vi "Test_ConstructTransport_InvalidRefnum_Error.vi"(8 "error in (no error)":errorcluster, 11 "TestCase in":refnum<class "TestFormattedStringBinding.lvclass">) -> (0 "error out":errorcluster, 3 "TestCase out":refnum<class "TestFormattedStringBinding.lvclass">)   [LabVIEW 2017, in "TestFormattedStringBinding.lvclass"]
uses:
  TestFormattedStringBinding.lvclass
  Source/Concrete/FormattedStringBinding/FormattedStringBinding.lvclass/FormattedStringBinding.ctl
  Source/Concrete/FormattedStringBinding/FormattedStringBinding.lvclass
  C:/Git/composed-transport/Source/Concrete/TerminalValueBinding/TerminalValueBinding.lvclass
  <vilib>/Utility/error.llb/Error Cluster From Error Code.vi
  Source/Concrete/TerminalValueBinding/Construct Terminal Value Binding.vi
panel:
  out "Return Error":errorcluster
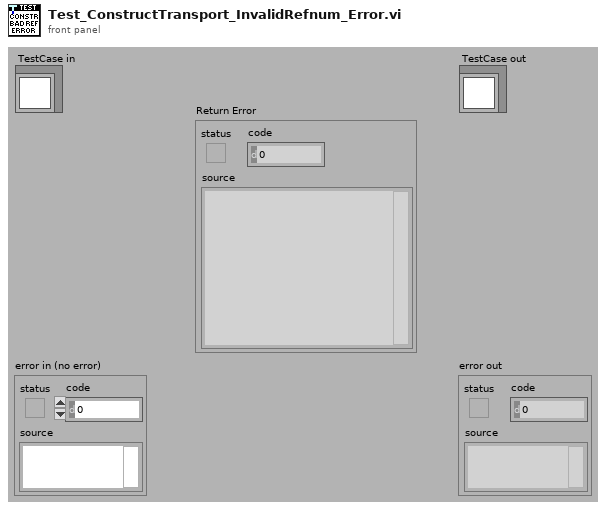
[diagram p1: front panel]
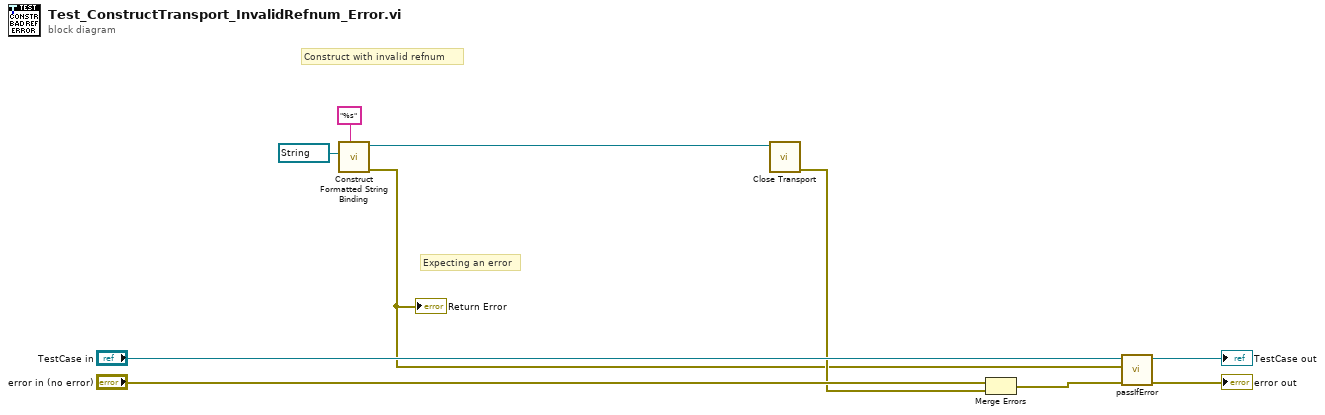
[diagram p0: block diagram]
diagram:
  # "Expecting an error"
  # "Construct with invalid refnum"
  n1 = call "Construct Formatted String Binding.vi"("Format String"="%s", "Str Refnum"=refnum<vi> refnum) -> ("error out"=w2:errorcluster, "FormattedStringBinding"=w3:refnum<class "FormattedStringBinding.lvclass">)  [unwired: 8 in]
  "Return Error" <- w2
  n2 = call-dynamic "Close Transport.vi"("ITransport in"=w3) -> ("error out"=w5:errorcluster)  [unwired: 10 in]
  n3 = Merge Errors("error in (no error)", w5) -> (w6:errorcluster)
  n4 = call-dynamic "passIfError.vi"("error in (no error)"=w6, "error"=w2, "TestCase in"="TestCase in") -> ("error out"=→"error out":errorcluster, "TestCase out"=→"TestCase out":refnum<class "TestFormattedStringBinding.lvclass">)  [unwired: 7 in]
